vi "Test Matrix Print.vi"() -> ()   [LabVIEW 2014, in "Arduino MatrixMath.lvlib"]
uses:
  <vilib>/Aledyne-TSXperts/Arduino Compatible Compiler for LabVIEW/addons/Arduino MatrixMath/Arduino MatrixMath.lvlib
panel:
  out "Error Out":errorcluster
  in  "Error In":errorcluster
  in  "A":sgl[](array[numeric])=[1.0, 2.0, 3.0, 4.0, 5.0, 6.0, 7.0, 8.0]
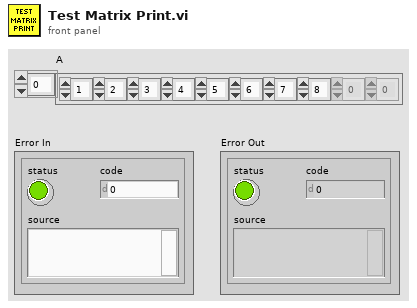
[diagram p1: front panel]
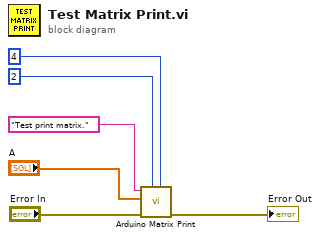
[diagram p0: block diagram]
diagram:
  n1 = call <vilib>:"Arduino Matrix Print.vi"("cols num."=u8 4, "rows num."=u8 2, "Error In"="Error In", "A"="A", "Label"="Test print matrix.") -> ("Error Out"=→"Error Out":errorcluster)  [unwired: 6 in]
